vi "PIDController.vi"(8 "error in (no error)":errorcluster, 11 "DAQ_QPT_Throlab in":refnum<class "DAQ_QPT_Throlab.lvclass">) -> (0 "error out":errorcluster, 3 "DAQ_QPT_Throlab out":refnum<class "DAQ_QPT_Throlab.lvclass">)   [LabVIEW 2020, in "DAQ_QPT_Throlab.lvlib" / "DAQ_QPT_Throlab.lvclass"]
uses:
  DAQ_QPT_Throlab.lvclass
  C:/Program Files/National Instruments/LabVIEW 2020/vi.lib/ActorFramework/Actor/Actor.lvclass
  DAQ_QPT_Throlab.lvclass/DAQ_QPT_Throlab.ctl
  <vilib>/ActorFramework/Actor/Actor.lvclass/Actor.ctl
  HAL Layer/Component/Interface/Communication Messages/SetStagePosition Msg/SetStagePosition Msg.lvclass/SetStagePosition Msg.ctl
  <vilib>/ActorFramework/Message Enqueuer/Message Enqueuer.lvclass/Message Enqueuer.ctl
  <vilib>/ActorFramework/Message Enqueuer/Enqueue.vi
  HAL Layer/Component/Interface/Communication Messages/SetStagePosition Msg/SetStagePosition Msg.lvclass
  C:/Program Files/National Instruments/LabVIEW 2020/vi.lib/ActorFramework/Message/Message.lvclass
  <vilib>/ActorFramework/Message Priority Queue/Priority Enqueue.vi
  <vilib>/ActorFramework/Actor/Actor.lvclass
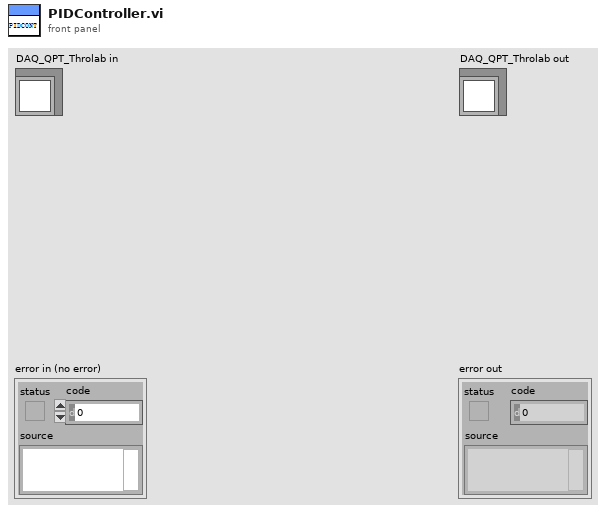
[diagram p1: front panel]
types:
  T1 = cluster{"Kp":dbl, "Ki":dbl, "Kd":dbl, "DeadZone(nm)":dbl}
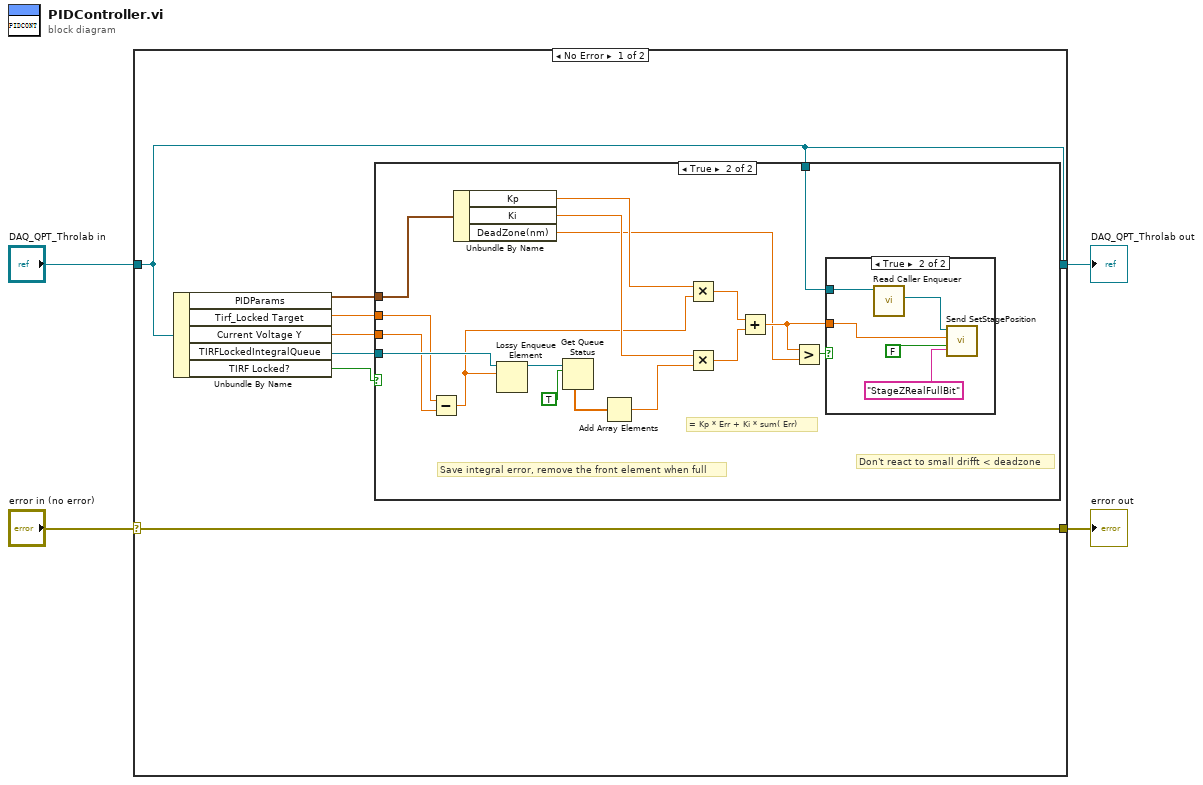
[diagram p0: block diagram]
diagram:
  n1 = case shown="No Error" "error in (no error)" {
    selector: "error in (no error)" -> [w11 w35]
    tunnel: [w11 w35] -> w3
    tunnel: [w6 w34] -> w1
    tunnel: "DAQ_QPT_Throlab in" -> [w6 w34]
    frame No Error {
      n2 = Unbundle By Name(w6) -> ("PIDParams"=w7:T1, "Tirf_Locked Target"=w9:dbl, "Current Voltage Y"=w8:dbl, "TIRFLockedIntegralQueue"=w10:refnum<queue>, "TIRF Locked?"=w5:bool)
      n3 = case shown="True" w5 {
        tunnel: w10 -> [_ w28]
        tunnel: w9 -> [_ w27]
        tunnel: w8 -> [_ w26]
        tunnel: w7 -> [_ w23]
        tunnel: w6 -> [_ w16]
        frame False {
        }
        frame True {
          # "Don't react to small drifft < deadzone"
          # "= Kp * Err + Ki * sum( Err)"
          # "Save integral error, remove the front element when full"
          n4 = Subtract(x=w27, y=w26) -> (x-y=w19:dbl)
          n5 = Unbundle By Name(w23) -> ("Kp"=w20:dbl, "Ki"=w22:dbl, "DeadZone(nm)"=w13:dbl)
          n6 = Lossy Enqueue Element(queue=w28, element=w19) -> (queue out=w25:refnum<queue>)  [unwired: 1 in, 3 out]
          n7 = Get Queue Status(queue=w25, return elements? (F)=TRUE) -> (elements=w24:dbl[])  [unwired: 1 in, 7 out]
          n8 = Add Array Elements(numeric array=w24) -> (sum=w21:dbl)
          n9 = Multiply(x=w20, y=w19) -> (x*y=w18:dbl)
          n10 = Multiply(x=w22, y=w21) -> (x*y=w17:dbl)
          n11 = Add(x=w18, y=w17) -> (x+y=w14:dbl)
          n12 = Greater?(x=w14, y=w13) -> (0:w12:bool)
          n13 = case shown="True" w12 {
            tunnel: w16 -> [_ w33]
            tunnel: w14 -> [_ w29]
            frame False {
            }
            frame True {
              n14 = call <vilib>:"Read Caller Enqueuer.vi"("Actor"=w33) -> ("Caller Enqueuer"=w32:refnum<class "Message Enqueuer.lvclass">)  [unwired: 10 in]
              n15 = call "Send SetStagePosition.vi"("Label"="StageZRealFullBit", "AbsPosition?"=FALSE, "Value"=w29, "Message Enqueuer"=w32) -> ()  [unwired: 6 in, 2 out]
            }
          }
        }
      }
    }
    frame Error {
    }
  }
  "error out" <- w3
  "DAQ_QPT_Throlab out" <- w1
